vi "build.epoch.vi"(10 "Time Unit":T1(ring), 11 "Time Series Name":string) -> (3 "ts.epochOfTimeUnit out":refnum<class "ts.epochOfTimeUnit.lvclass">)   [LabVIEW 2020, in "ts.epochOfTimeUnit.lvclass"]
uses:
  ts.epochOfTimeUnit.lvclass
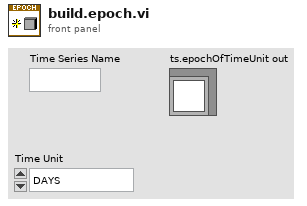
[diagram p1: front panel]
types:
  T1 = enum16{"DAYS", "HOURS", "MINUTES", "SECONDS", "MILLISECONDS", "MICROSECONDS", "NANOSECONDS", "PICOSECONDS"}
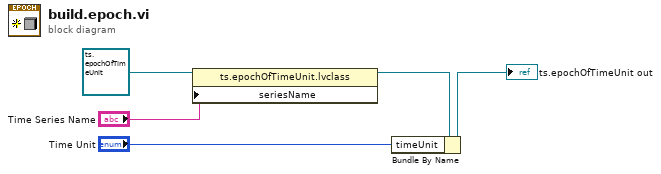
[diagram p0: block diagram]
diagram:
  n1 = property class="ts.epochOfTimeUnit.lvclass"(reference=refnum<class "ts.epochOfTimeUnit.lvclass"> refnum ("ts.epochOfTimeUnit in"), "seriesName"="Time Series Name") -> (reference out=w3:refnum<class "ts.epochOfTimeUnit.lvclass">)  [unwired: 1 in, 1 out]
  n2 = Bundle By Name(cluster=w3, "timeUnit"="Time Unit") -> (→"ts.epochOfTimeUnit out":refnum<class "ts.epochOfTimeUnit.lvclass">)
